vi "shift_below_1.vi"(4 "ready for output":bool, 5 "input valid":bool, 7 "input":fxp<+/-,64,32>) -> (0 "ready for input":bool=TRUE, 1 "output valid":bool, 2 "shifted":fxp<+/-,64,32>, 3 "count":i16)   [LabVIEW 2018]
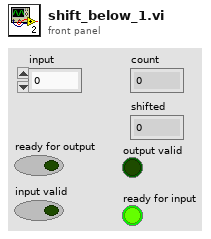
[diagram p1: front panel]
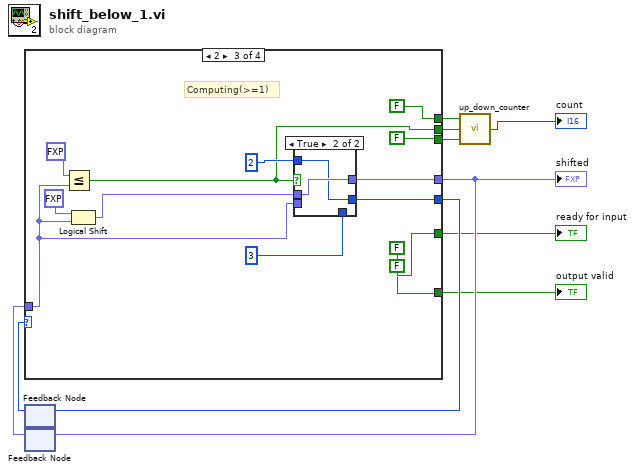
[diagram p0: block diagram]
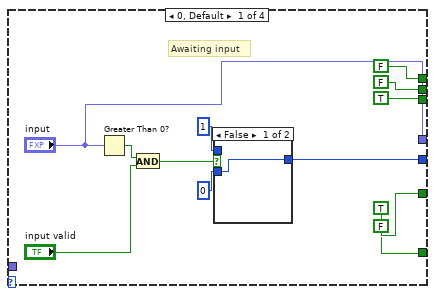
[diagram p2: hidden frame]
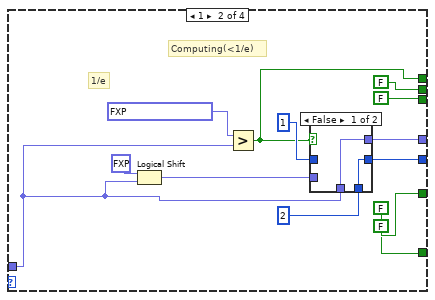
[diagram p4: hidden frame]
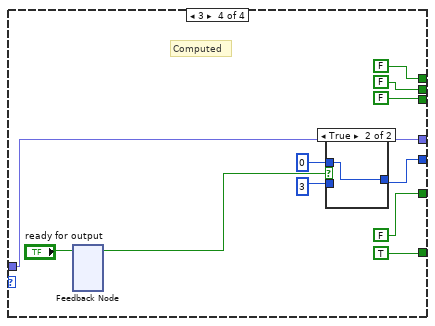
[diagram p7: hidden frame]
diagram:
  n1 = feedback #1() -> (w9:u8)  [unwired: 1 in]
  n2 = feedback #2() -> (w7:fxp<+/-,64,32>)  [unwired: 1 in]
  n3 = case shown="2" w9 {
    tunnel: [w12 w30 w42 w62] -> w10
    tunnel: ["input" w31 w48 w66] -> w8
    tunnel: w7 -> [_ w26 w45 w66]
    tunnel: [TRUE FALSE FALSE FALSE] -> w6
    tunnel: [FALSE FALSE w43 FALSE] -> w5
    tunnel: [FALSE w25 FALSE FALSE] -> w4
    tunnel: [TRUE FALSE FALSE FALSE] -> w3
    tunnel: [FALSE FALSE FALSE TRUE] -> w2
    frame 0, Default {
      # "Awaiting input"
      n4 = Greater Than 0?(x="input") -> (x > 0?=w22:bool)
      n5 = And(x=w22, y="input valid") -> (x .and. y?=w11:bool)
      n6 = case shown="False" w11 {
        tunnel: u8 1 -> [_ w24]
        tunnel: u8 0 -> [w23 _]
        tunnel: [w23 w24] -> w12
        frame False {
        }
        frame True {
        }
      }
    }
    frame 1 {
      # "1/e"
      # "Computing(<1/e)"
      n7 = Logical Shift(y=fxp<+,1,1> 1.0, x=w26) -> (x << y=w27:fxp<+/-,64,32>)
      n8 = Greater?(x=fxp<+,15,-1> 0.367889404296875, y=w26) -> (0:w25:bool)
      n9 = case shown="False" w25 {
        tunnel: [w38 w40] -> w31
        tunnel: [w39 w41] -> w30
        tunnel: u8 1 -> [_ w41]
        tunnel: u8 2 -> [w39 _]
        tunnel: w27 -> [_ w40]
        tunnel: w26 -> [w38 _]
        frame False {
        }
        frame True {
        }
      }
    }
    frame 2 {
      # "Computing(>=1)"
      n10 = Less Or Equal?(x=fxp<+,1,1> 1.0, y=w45) -> (x <= y?=w43:bool)
      n11 = Logical Shift(y=fxp<+/-,1,1> -1.0, x=w45) -> (x << y=w44:fxp<+/-,64,32>)
      n12 = case shown="True" w43 {
        tunnel: [w55 w58] -> w48
        tunnel: u8 2 -> [_ w57]
        tunnel: u8 3 -> [w56 _]
        tunnel: w45 -> [w55 _]
        tunnel: w44 -> [_ w58]
        tunnel: [w56 w57] -> w42
        frame False {
        }
        frame True {
        }
      }
    }
    frame 3 {
      # "Computed"
      n13 = feedback #3() -> (w59:bool)  [unwired: 1 in]
      n14 = feedback-in #3("ready for output") -> ()
      n15 = case shown="True" w59 {
        tunnel: u8 0 -> [_ w71]
        tunnel: u8 3 -> [w70 _]
        tunnel: [w70 w71] -> w62
        frame False {
        }
        frame True {
        }
      }
    }
  }
  "output valid" <- w2
  "ready for input" <- w3
  "shifted" <- w8
  n16 = feedback-in #1(w10) -> ()
  n17 = feedback-in #2(w8) -> ()
  n18 = call "up_down_counter.vi"("reset"=w6, "up"=w5, "down"=w4) -> ("Value"=→"count":i16)
